vi "Set Magnetometer via DAC (SubVI).vi"(8 "error constant":errorcluster, 9 "DAQmx":tag, 10 "M[mgauss]":ext, 11 "Axis":T1(ring)) -> (0 "error constant 2":errorcluster)   [LabVIEW 2017]
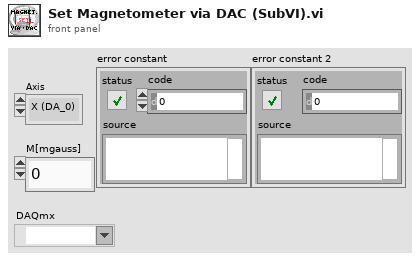
[diagram p1: front panel]
types:
  T1 = enum16{"X (DA_0)", "Y (DA_1)", "Z (DA_2)", "DA_3"}
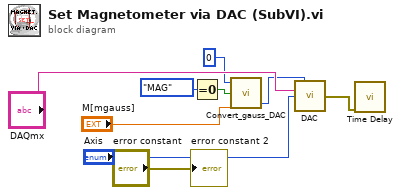
[diagram p0: block diagram]
diagram:
  n1 = Equal To 0?(x=enum16{"MAG", "DAC"}."MAG" ("Enum 2")) -> (x = 0?=w4:bool)
  n2 = call "Convert_gauss_DAC.vi"("M[mgauss]in"="M[mgauss]", "DAC_F"=w4, "DB0-11DAC"=u16 0 ("DAC")) -> ("DB0-11 out"=w7:u16)  [unwired: 1 in, 1 out]
  n3 = call "DAC.vi"("DB0-11 2"=w7, "device name"="DAQmx", "Enum 2"="Axis") -> ("error out"=w1:errorcluster)  [unwired: 12 in]
  n4 = call "Time Delay"("error in (no error)"=w1) -> ()  [unwired: 10 in, 1 out]
  "error constant 2" <- "error constant"
